vi "from string 1.0.vi"(8 "error in (no error)":errorcluster, 10 "data":string, 11 "E2E configuration in":refnum<class "E2E Tag Exchange configuration.lvclass">) -> (0 "error out":errorcluster, 3 "E2E configuration out":refnum<class "E2E Tag Exchange configuration.lvclass">)   [LabVIEW 2015, in "E2E Tag Exchange configuration.lvclass"]
uses:
  E2E Tag Exchange configuration.lvclass
  Runtime Implementation.ctl
  <vilib>/NI/Tag Bus Module Framework/channel/TBM channel.lvclass
  E2E Tag Exchange configuration.lvclass/E2E Tag Exchange configuration.ctl
  <vilib>/NI/Configuration Framework/serializable configuration/NISE_CEF_serializable configuration.lvclass
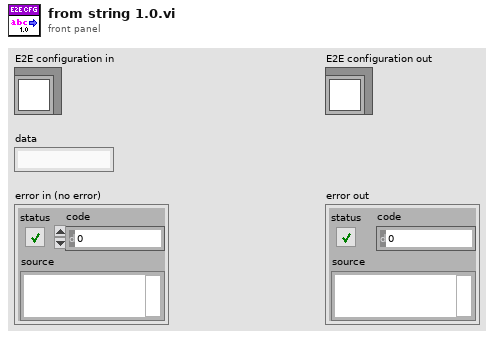
[diagram p1: front panel]
types:
  T1 = typedef "E2E Tag Exchange configuration.lvclass/Runtime Implementation.ctl" = enum16{"RT FIFO", "UDP"}
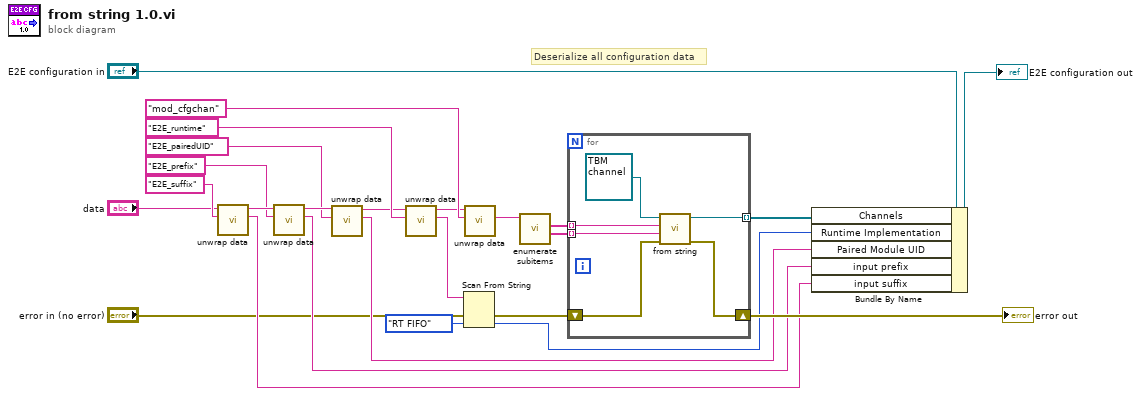
[diagram p0: block diagram]
diagram:
  # "Deserialize all configuration data"
  n1 = call <vilib>:"unwrap data.vi"("identifier"="E2E_suffix", "data to unwrap"="data") -> ("unwrapped data"=w6:string, "remaining string"=w8:string)  [unwired: 8 in]
  n2 = call <vilib>:"unwrap data.vi"("identifier"="E2E_prefix", "data to unwrap"=w8) -> ("unwrapped data"=w9:string, "remaining string"=w7:string)  [unwired: 8 in]
  n3 = call <vilib>:"unwrap data.vi"("identifier"="E2E_pairedUID", "data to unwrap"=w7) -> ("unwrapped data"=w10:string, "remaining string"=w11:string)  [unwired: 8 in]
  n4 = call <vilib>:"unwrap data.vi"("identifier"="E2E_runtime", "data to unwrap"=w11) -> ("unwrapped data"=w14:string, "remaining string"=w16:string)  [unwired: 8 in]
  n5 = Scan From String(input string=w14, error in="error in (no error)", default 1=Runtime_Implementation."RT FIFO" ("Runtime Implementation")) -> (error out=w15:errorcluster, output 1=w12:T1)  [unwired: 2 in, 2 out]
  n6 = call <vilib>:"unwrap data.vi"("identifier"="mod_cfgchan", "data to unwrap"=w16) -> ("unwrapped data"=w24:string)  [unwired: 8 in, 1 out]
  n7 = call <vilib>:"enumerate subitems.vi"("data to enumerate"=w24) -> ("associated data"=w23:string[], "discovered subitems"=w22:string[])  [unwired: 8 in, 1 out]
  n8 = for {
    shift-right: [w31] -> w25
    shift-left: w15 -> [w30]
    tunnel: w22 -> [w29] mode=indexing
    tunnel: w23 -> [w28] mode=indexing
    tunnel: [w26] -> w18 mode=indexing
    n9 = call-dynamic "from string.vi"("error in"=w30, "channel data"=w28, "identifier"=w29, "channel in"=refnum<class "TBM channel.lvclass"> refnum) -> ("error out"=w31:errorcluster, "channel out"=w26:refnum<class "TBM channel.lvclass">)  [unwired: 6 in]
  }
  "error out" <- w25
  n10 = Bundle By Name(cluster="E2E configuration in", "Channels"=w18, "Runtime Implementation"=w12, "Paired Module UID"=w10, "input prefix"=w9, "input suffix"=w6) -> (→"E2E configuration out":refnum<class "E2E Tag Exchange configuration.lvclass">)
